vi "Get Class.vi"(8 "error in (no error)":errorcluster, 11 "UDP in":refnum<class "UDP Transceiver.lvclass">) -> (0 "error out":errorcluster, 2 "class":string, 3 "UDP out":refnum<class "UDP Transceiver.lvclass">)   [LabVIEW 2017, in "UDP Transceiver.lvlib" / "UDP Transceiver.lvclass"]
uses:
  UDP Transceiver.lvclass
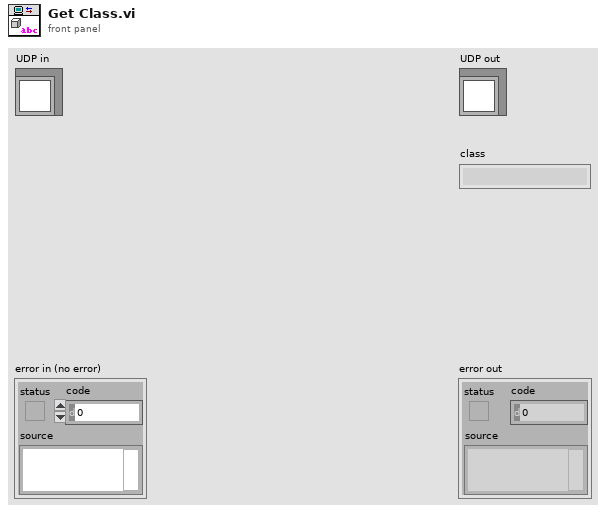
[diagram p1: front panel]
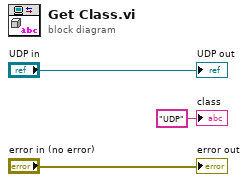
[diagram p0: block diagram]
diagram:
  "error out" <- "error in (no error)"
  "UDP out" <- "UDP in"
  "class" <- "UDP" ("class")
